vi "SignalGenerator_8_125Mhz.vi"(10 "Phase":fxp<+,64,64>[](array[numeric])=[0.0, 0.0, 0.0, 0.0, 0.0, 0.0, 0.0, 0.0], 11 "reset":bool) -> (1 "Sine out":fxp<+/-,16,0>[](array[numeric]), 2 "Cosine out":fxp<+/-,16,0>[](array[numeric]))   [LabVIEW 2013]
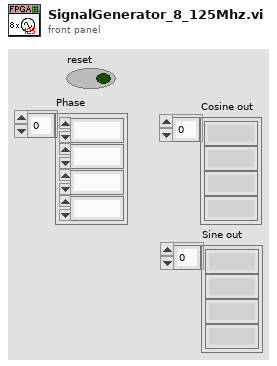
[diagram p1: front panel]
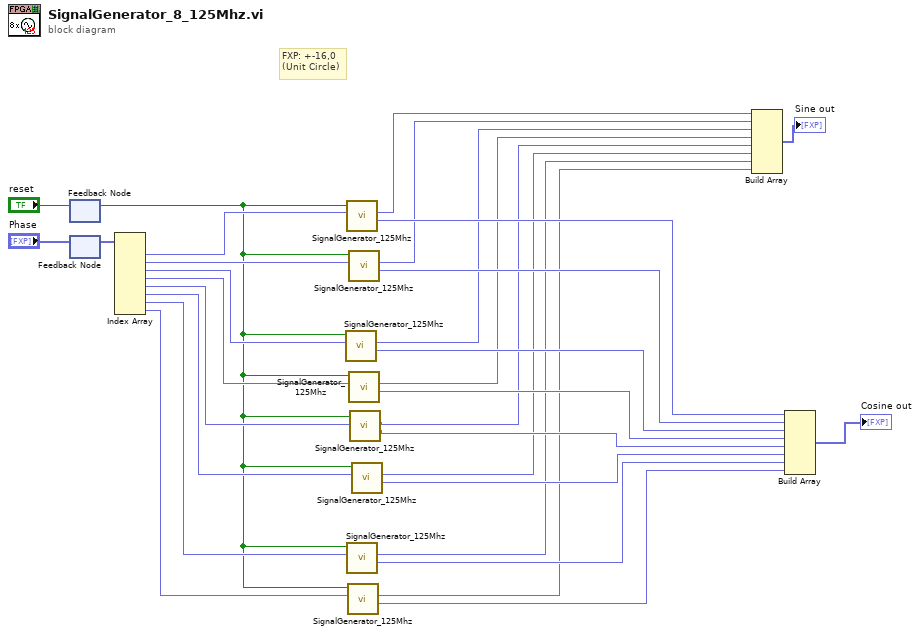
[diagram p0: block diagram]
diagram:
  # "FXP: +-16,0\n(Unit Circle)"
  n1 = feedback #1() -> (w15:bool)  [unwired: 1 in]
  n2 = feedback-in #1("reset") -> ()
  n3 = feedback #2() -> (w27:fxp<+,64,64>[])  [unwired: 1 in]
  n4 = feedback-in #2("Phase") -> ()
  n5 = Index Array(array=w27) -> (element #1=w25:fxp<+,64,64>, element #2=w16:fxp<+,64,64>, element #3=w17:fxp<+,64,64>, element #4=w18:fxp<+,64,64>, element #5=w19:fxp<+,64,64>, element #6=w20:fxp<+,64,64>, element #7=w21:fxp<+,64,64>, element #8=w22:fxp<+,64,64>)  [unwired: 8 in]
  n6 = call "SignalGenerator_125Mhz.vi"("phase"=w17, "Reset"=w15) -> ("Cos"=w11:fxp<+/-,16,0>, "Sin"=w12:fxp<+/-,16,0>)  [unwired: 7 in, 1 out]
  n7 = call "SignalGenerator_125Mhz.vi"("phase"=w25, "Reset"=w15) -> ("Cos"=w23:fxp<+/-,16,0>, "Sin"=w24:fxp<+/-,16,0>)  [unwired: 7 in, 1 out]
  n8 = call "SignalGenerator_125Mhz.vi"("phase"=w21, "Reset"=w15) -> ("Cos"=w3:fxp<+/-,16,0>, "Sin"=w4:fxp<+/-,16,0>)  [unwired: 7 in, 1 out]
  n9 = call "SignalGenerator_125Mhz.vi"("phase"=w22, "Reset"=w15) -> ("Cos"=w1:fxp<+/-,16,0>, "Sin"=w2:fxp<+/-,16,0>)  [unwired: 7 in, 1 out]
  n10 = call "SignalGenerator_125Mhz.vi"("phase"=w16, "Reset"=w15) -> ("Cos"=w13:fxp<+/-,16,0>, "Sin"=w14:fxp<+/-,16,0>)  [unwired: 7 in, 1 out]
  n11 = call "SignalGenerator_125Mhz.vi"("phase"=w18, "Reset"=w15) -> ("Cos"=w9:fxp<+/-,16,0>, "Sin"=w10:fxp<+/-,16,0>)  [unwired: 7 in, 1 out]
  n12 = call "SignalGenerator_125Mhz.vi"("phase"=w19, "Reset"=w15) -> ("Cos"=w7:fxp<+/-,16,0>, "Sin"=w8:fxp<+/-,16,0>)  [unwired: 7 in, 1 out]
  n13 = call "SignalGenerator_125Mhz.vi"("phase"=w20, "Reset"=w15) -> ("Cos"=w5:fxp<+/-,16,0>, "Sin"=w6:fxp<+/-,16,0>)  [unwired: 7 in, 1 out]
  n14 = Build Array(w24, w14, w12, w10, w8, w6, w4, w2) -> (→"Sine out":fxp<+/-,16,0>[])
  n15 = Build Array(w23, w13, w11, w9, w7, w5, w3, w1) -> (→"Cosine out":fxp<+/-,16,0>[])
